vi "tune_motors.vi"(9 "time":dbl format="%0.2f") -> (3 "desired Tensions array":dbl[](array[numeric]))   [LabVIEW 2017]
uses:
  <vilib>/ptbypt/NI_PtbyPt.lvlib
panel:
  in  "index motor":i32
  in  "F(N)":dbl
  in  "phase":dbl=200.0
  in  "freq":dbl=0.5
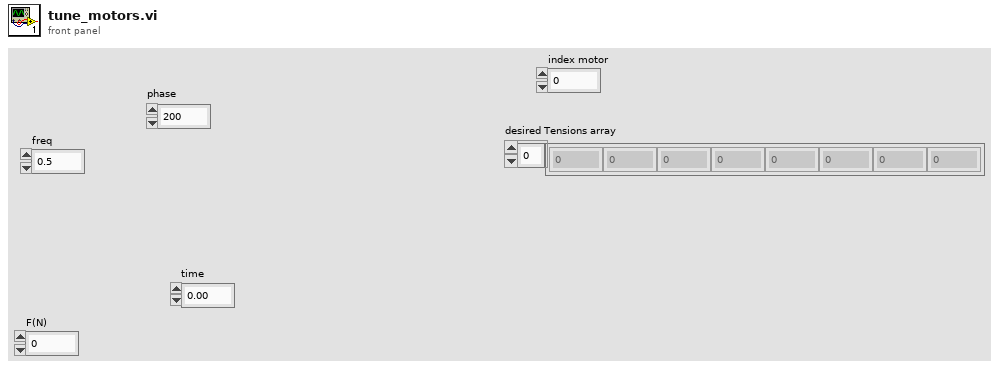
[diagram p1: front panel]
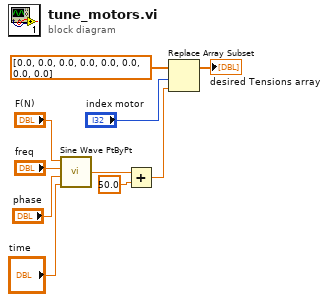
[diagram p0: block diagram]
diagram:
  n1 = call <vilib>:"Sine Wave PtByPt.vi"("time"="time", "phase"="phase", "frequency"="freq", "amplitude"="F(N)") -> ("sine wave"=w3:dbl)
  n2 = Add(x=w3, y=50.0) -> (x+y=w2:dbl)
  n3 = Replace Array Subset(array=dbl[] [0.0, 0.0, 0.0, 0.0, 0.0, 0.0, 0.0, 0.0], new element=w2, index="index motor") -> (→"desired Tensions array":dbl[])
